vi "GetControlsRefFromVIRef.vi"(0 "VI Reference In":refnum<vi>, 11 "Error In":errorcluster) -> (4 "VI Reference Out":refnum<vi>, 8 "Controls[]":refnum<vi>[](array[refnum]), 15 "Error Out":errorcluster)   [LabVIEW 2016, in "Drona.lvlib" / "GetControlRef.lvlib"]
doc: "<b>Gives the reference of controls in the VI.</b>"
uses:
  GetControlRef.lvlib
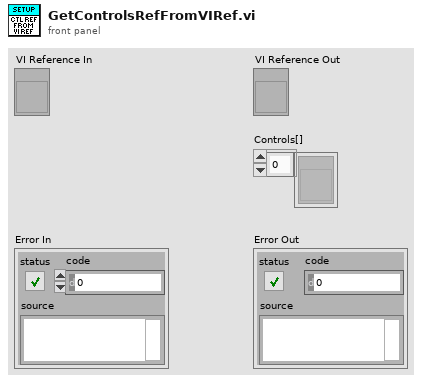
[diagram p1: front panel]
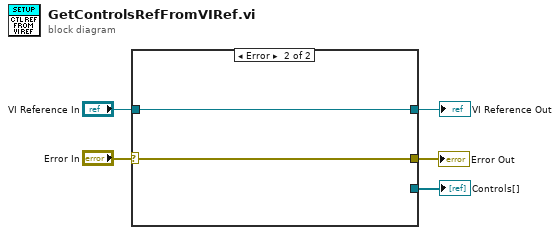
[diagram p0: block diagram]
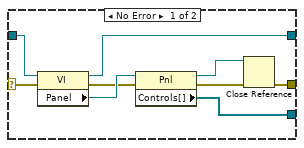
[diagram p2: hidden frame]
diagram:
  n1 = case shown="Error" "Error In" {
    selector: "Error In" -> [w7 w15]
    tunnel: "VI Reference In" -> [w14 w16]
    tunnel: [w11 w16] -> w4
    tunnel: [w10 _] -> w3
    tunnel: [w9 w15] -> w2
    frame No Error {
      n2 = property class="VI"(reference=w14, error in=w7) -> (reference out=w11:refnum<vi>, error out=w12:errorcluster, "Panel"=w13:refnum<vi>)
      n3 = property class="Pnl"(reference=w13, error in=w12) -> (reference out=w8:refnum<vi>, error out=w6:errorcluster, "Controls[]"=w10:refnum<vi>[])
      n4 = Close Reference(reference=w8, error in (no error)=w6) -> (error out=w9:errorcluster)
    }
    frame Error {
    }
  }
  "VI Reference Out" <- w4
  "Controls[]" <- w3
  "Error Out" <- w2
